vi "Analysator reduzieren.vi"(8 "error in (no error)":errorcluster caption="Fehler (Eingang, kein Fehler)", 11 "Kombinationsfeld (Eingang)":refnum<vi>) -> (0 "error out":errorcluster caption="Fehler (Ausgang)", 2 "Wert":T1="N2", 3 "Strings And Values[]":T2)   [LabVIEW 2020, in "System Einstellungen V2.lvlib"]
uses:
  System Einstellungen V2.lvlib
  <vilib>/Utility/miscctls.llb/LVComboBoxStrsAndValuesArrayTypeDef.ctl
  Analysatoren.ctl
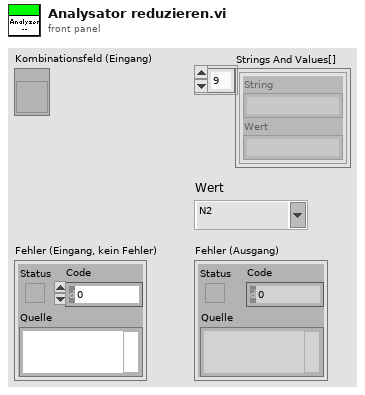
[diagram p1: front panel]
types:
  T1 = typedef "System Einstellungen V2.lvlib/Analysatoren.ctl" = string
  T2 = typedef "LVComboBoxStrsAndValuesArrayTypeDef.ctl" = cluster{"String":string, "Value":string}[]
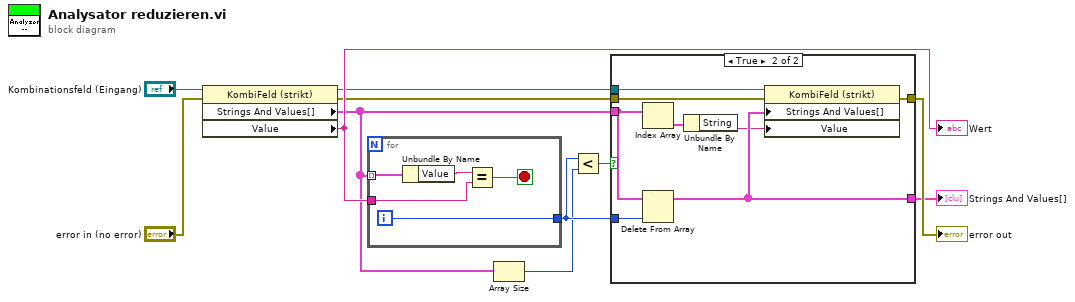
[diagram p0: block diagram]
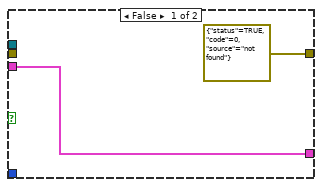
[diagram p2: hidden frame]
diagram:
  n1 = property class="KombiFeld (strikt)"(reference="Kombinationsfeld (Eingang)", error in="error in (no error)") -> (reference out=w8:refnum<vi>, error out=w7:errorcluster, "Strings And Values[]"=w4:T2, "Value"=w9:T1)
  "Wert" <- w9
  n2 = for {
    tunnel: w4 -> [w16] mode=indexing
    tunnel: w9 -> [w15]
    tunnel: [w12] -> w2
    i -> [w12]
    stop <- w13 stop-if-true
    n3 = Unbundle By Name(w16) -> ("Value"=w14:string)
    n4 = Equal?(x=w14, y=w15) -> (x = y?=w13:bool)
  }
  n5 = Array Size(array=w4) -> (size(s)=w1:i32)
  n6 = Less?(x=w2, y=w1) -> (x < y?=w3:bool)
  n7 = case shown="True" w3 {
    tunnel: w2 -> [_ w26]
    tunnel: w8 -> [_ w25]
    tunnel: w7 -> [_ w24]
    tunnel: [errorcluster {"status"=TRUE, "code"=0, "source"="not found"} ("error out") w23] -> w6
    tunnel: [w18 w22] -> w5
    tunnel: w4 -> [w18 w21]
    frame False {
    }
    frame True {
      n8 = Index Array(array=w21) -> (element=w20:cluster{"String":string, "Value":string})  [unwired: 1 in]
      n9 = Delete From Array(array=w21, index=w26) -> (array with subset deleted=w22:T2)  [unwired: 1 in, 1 out]
      n10 = Unbundle By Name(w20) -> ("String"=w19:string)
      n11 = property class="KombiFeld (strikt)"(reference=w25, error in=w24, "Strings And Values[]"=w22, "Value"=w19) -> (error out=w23:errorcluster)  [unwired: 1 out]
    }
  }
  "error out" <- w6
  "Strings And Values[]" <- w5
